vi "Transfer_data.vi"(8 "error in (no error)":errorcluster, 9 "Start":dbl, 10 "Points":u32=4096, 11 "Initialize_card in":refnum<class "Initialize_card.lvclass">) -> (0 "error out":errorcluster, 1 "Data in Volts":dbl[](array[numeric]), 3 "Initialize_card out":refnum<class "Initialize_card.lvclass">)   [LabVIEW 2015, in "Initialize_card.lvclass"]
uses:
  Initialize_card.lvclass
panel:
  out "Waveform Graph":cluster{dbl, dbl, "Data in Volts":dbl[]}(graph)
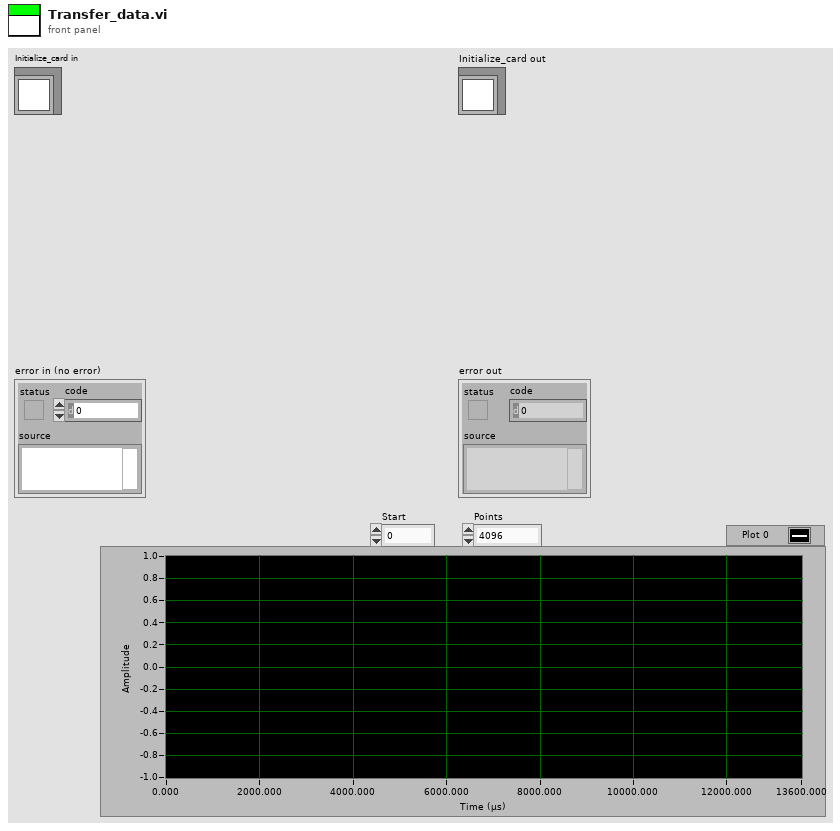
[diagram p1: front panel]
types:
  T1 = cluster{"Handle":u32, "Sample size":u32, "Resolution":i32, "Offset":i32, "Channels":u32, "Boards":u32}
  T2 = cluster{"Handle":u32, "Sample Size":u32, "Resolution":i32, "Offset":i32, "Channels":u32, "Boards":u32}
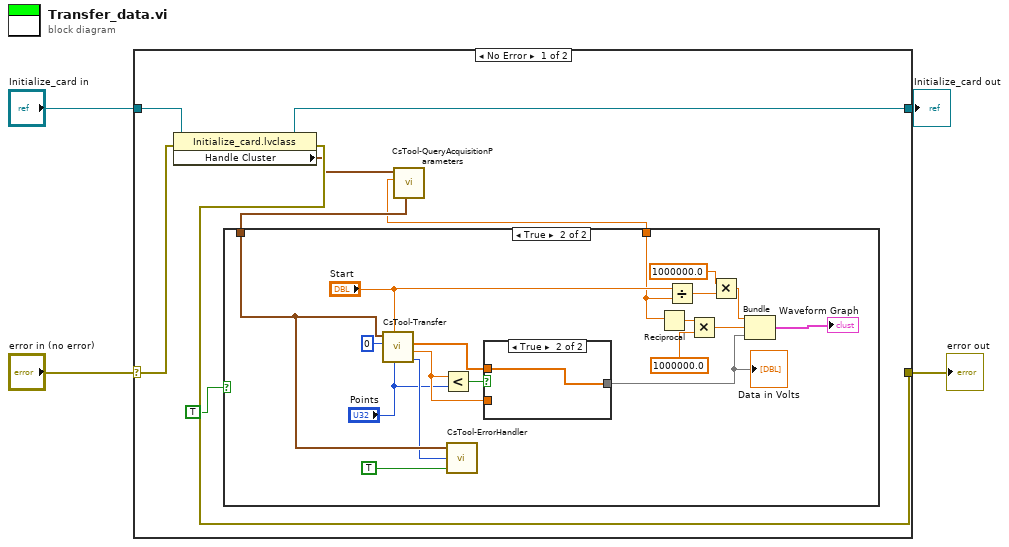
[diagram p0: block diagram]
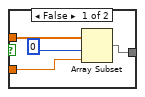
[diagram p3: hidden frame]
diagram:
  n1 = case shown="No Error" "error in (no error)" {
    selector: "error in (no error)" -> [w11 w37]
    tunnel: [w10 w37] -> w3
    tunnel: [w9 w36] -> w1
    tunnel: "Initialize_card in" -> [w12 w36]
    frame No Error {
      n2 = property class="Initialize_card.lvclass"(reference=w12, error in=w11) -> (reference out=w9:refnum<class "Initialize_card.lvclass">, error out=w10:errorcluster, "Handle Cluster"=w8:T1)
      n3 = call <userlib>:"CsTool-QueryAcquisitionParameters.vi"("Handle Cluster"=w8) -> ("Output Handle Cluster"=w7:T2, "Sample Rate"=w6:dbl)  [unwired: 9 out]
      n4 = case shown="True" TRUE {
        tunnel: w6 -> [_ w22]
        tunnel: w7 -> [_ w21]
        frame False {
        }
        frame True {
          n5 = call <userlib>:"CsTool-Transfer.vi"("Length (4096)"="Points", "Start (0)"="Start", "Channel (0)"=u16 0, "Handle Cluster"=w21) -> ("Error Code"=w16:i32, "Actual Length"=w18:dbl, "Data in Volts"=w17:dbl[])  [unwired: 2 in, 1 out]
          n6 = Less?(x=w18, y="Points") -> (x < y?=w19:bool)
          n7 = call <userlib>:"CsTool-ErrorHandler.vi"("StopOnError (true)"=TRUE, "Error Code"=w16, "Handle Cluster"=w21) -> ()  [unwired: 1 out]
          n8 = case shown="True" w19 {
            tunnel: w17 -> [w34 w35]
            tunnel: w18 -> [w32 _]
            tunnel: [w31 w35] -> w25
            frame False {
              n9 = Array Subset(array=w34, index=0, length=w32) -> (w31:dbl[])
            }
            frame True {
            }
          }
          "Data in Volts" <- w25
          n10 = Reciprocal(x=w22) -> (1/x=w27:dbl)
          n11 = Divide(x="Start", y=w22) -> (x/y=w30:dbl)
          n12 = Multiply(x=w27, y=1000000.0) -> (x*y=w29:dbl)
          n13 = Multiply(x=1000000.0, y=w30) -> (x*y=w20:dbl)
          n14 = Bundle(w20, w29, "Data in Volts"=w25) -> (→"Waveform Graph":cluster{dbl, dbl, "Data in Volts":dbl[]})  [unwired: 1 in]
        }
      }
    }
    frame Error {
    }
  }
  "error out" <- w3
  "Initialize_card out" <- w1
